vi "test_mode_calculator.vi"(0 "Mode":T2(ring), 1 "Hi-Pot test time":dbl min=0.0 format="%.2f", 2 "GB test time":dbl min=0.0 format="%.2f", 3 "Delay":dbl min=0.0 format="%.2f") -> (6 "Mode parameters":T1 {"delay" format="%.2f"; "test time" format="%.2f"; "overlap" format="%.2f"; "T2 test" format="%.2f"; "T1 test" format="%.2f"})   [LabVIEW 2015]
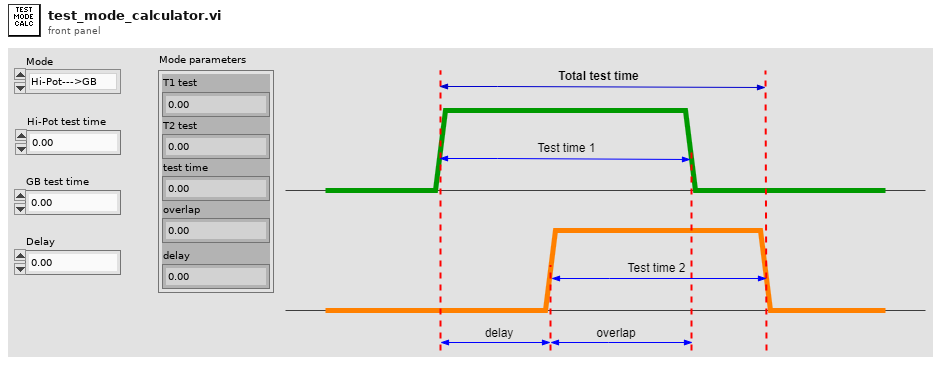
[diagram p1: front panel]
types:
  T1 = cluster{"T1 test":dbl, "T2 test":dbl, "overlap":dbl, "test time":dbl, "delay":dbl}
  T2 = enum16{"Hi-Pot--->GB", "GB--->Hi-Pot", "Hi-Pot only", "GB only"}
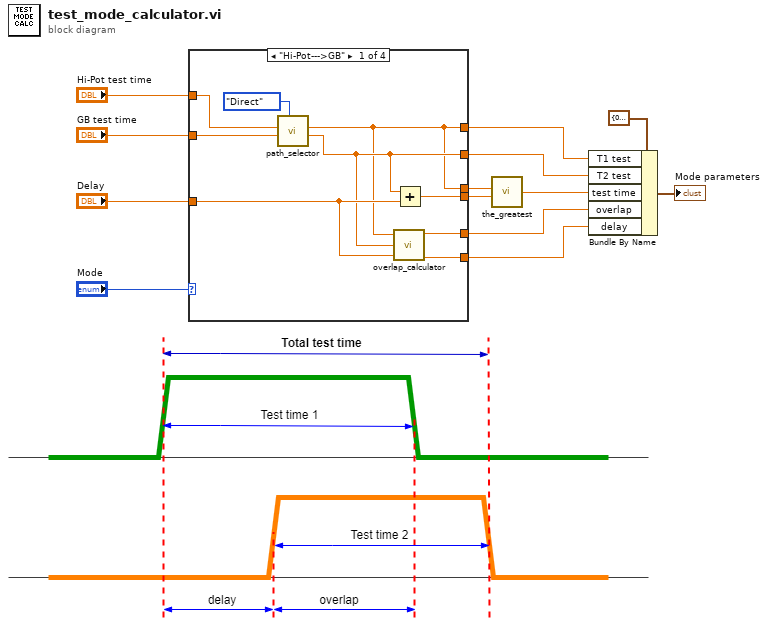
[diagram p0: block diagram]
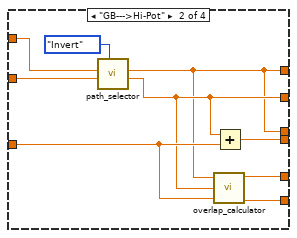
[diagram p2: hidden frame]
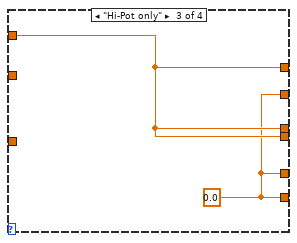
[diagram p3: hidden frame]
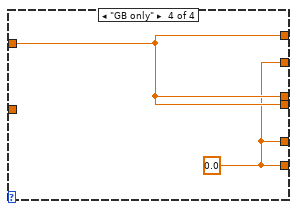
[diagram p4: hidden frame]
diagram:
  n1 = case shown="\"Hi-Pot--->GB\"" "Mode" {
    tunnel: "Hi-Pot test time" -> [w17 w28 w33 _]
    tunnel: "GB test time" -> [w16 w27 _ w35]
    tunnel: "Delay" -> [w20 w25 _ _]
    tunnel: [w22 w31 w33 w35] -> w13
    tunnel: [w14 w23 w33 w35] -> w12
    tunnel: [w14 w23 w33 w35] -> w6
    tunnel: [w15 w24 w32 w34] -> w7
    tunnel: [w21 w30 w32 w34] -> w4
    tunnel: [w19 w29 w32 w34] -> w3
    frame "Hi-Pot--->GB" {
      n2 = call "path_selector.vi"("Selector"=enum16{"Direct", "Invert"}."Direct", "GB test time"=w16, "Hi-Pot test time"=w17) -> ("T2"=w15:dbl, "T1"=w14:dbl)  [unwired: 7 in]
      n3 = call "overlap_calculator.vi"("T1"=w14, "T2"=w15, "D"=w20) -> ("overlap"=w21:dbl, "delay"=w19:dbl)  [unwired: 6 in]
      n4 = Add(x=w15, y=w20) -> (x+y=w22:dbl)
    }
    frame "GB--->Hi-Pot" {
      n5 = call "path_selector.vi"("Selector"=enum16{"Direct", "Invert"}."Invert", "GB test time"=w27, "Hi-Pot test time"=w28) -> ("T2"=w24:dbl, "T1"=w23:dbl)  [unwired: 7 in]
      n6 = call "overlap_calculator.vi"("T1"=w23, "T2"=w24, "D"=w25) -> ("overlap"=w30:dbl, "delay"=w29:dbl)  [unwired: 6 in]
      n7 = Add(x=w24, y=w25) -> (x+y=w31:dbl)
    }
    frame "Hi-Pot only" {
      w32 = 0.0
    }
    frame "GB only" {
      w34 = 0.0
    }
  }
  n8 = call "the_greatest.vi"("T1"=w12, "T2 + D"=w13) -> ("max"=w5:dbl)  [unwired: 6 in]
  n9 = Bundle By Name(cluster=T1 {"T1 test"=0.0, "T2 test"=0.0, "overlap"=0.0, "test time"=0.0, "delay"=0.0} ("Mode parameters"), "T1 test"=w6, "T2 test"=w7, "test time"=w5, "overlap"=w4, "delay"=w3) -> (→"Mode parameters":T1)
